vi "Get Folder.vi"(8 "error in":errorcluster) -> (0 "error out":errorcluster, 3 "dup path":path)   [LabVIEW 2014, in "Logger.lvlib"]
uses:
  Logger.lvlib
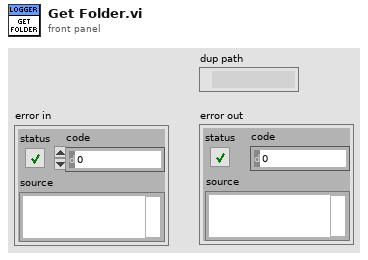
[diagram p1: front panel]
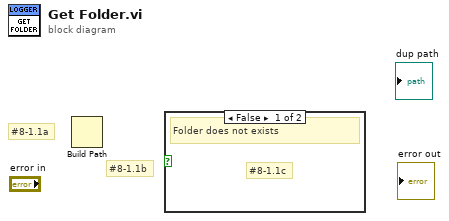
[diagram p0: block diagram]
diagram:
  # "#8-1.1b"
  # "#8-1.1a"
  n1 = Build Path() -> ()  [unwired: 2 in, 1 out]
  n2 = case shown="False" {
    selector: _ -> [_ _]
    frame False {
      # "#8-1.1c"
      # "Folder does not exists"
    }
    frame True {
      # "Folder exists"
    }
  }
